vi "GUI_DG645_1.0.0.vi"() -> ()   [LabVIEW 2020]
uses:
  Device Drivers/DG645/subVIs/TriggerSource_TypDef.ctl
  Device Drivers/DG645/subVIs/Inhibit_TypDef.ctl
  Device Drivers/shared/OnOffTypeDef.ctl
  Device Drivers/DG645/subVIs/polarity_TypDEf.ctl
  DelayControl_For Multiple Channels.ctl
  Device Drivers/DG645/subVIs/channels_TypDef.ctl
  DelayControl2.ctl
  Device Drivers/DG645/subVIs/saveLocal_TypDef.ctl
panel:
  in  "time to wait (TCP) 2":i32=10
  in  "plot":bool=TRUE
  out "ratio(h)":bool
  out "fixsize":bool
  in  "shotnumber":i32
  out "error (h)":bool
  out "Device Name (h)":string="StagingDG645 1"
  in  "Main Tap":T1(tab)
  in  "Delay.Ch T1":T2={"Channel"="T1", "Linked"=enum."T0", "Delay"=0.03} {"Delay" format="%+.12f"}
  in  "Delay.Ch T0":T2={"Channel"="T0", "Linked"=enum."T0", "Delay"=0.0} {"Delay" format="%+.12f"}
  in  "Delay.Ch H":T2={"Channel"="H", "Linked"=enum."G", "Delay"=0.03} {"Delay" format="%+.12f"}
  in  "Delay.Ch G":T2={"Channel"="G", "Linked"=enum."T0", "Delay"=0.0} {"Delay" format="%+.12f"}
  in  "Delay.Ch F":T2={"Channel"="F", "Linked"=enum."E", "Delay"=0.03} {"Delay" format="%+.12f"}
  in  "Delay.Ch E":T2={"Channel"="E", "Linked"=enum."T0", "Delay"=0.0} {"Delay" format="%+.12f"}
  in  "Delay.Ch D":T2={"Channel"="D", "Linked"=enum."C", "Delay"=0.03} {"Delay" format="%+.12f"}
  in  "Delay.Ch C":T2={"Channel"="C", "Linked"=enum."T0", "Delay"=0.0} {"Delay" format="%+.12f"}
  in  "Delay.Ch B":T2={"Channel"="B", "Linked"=enum."A", "Delay"=0.03} {"Delay" format="%+.12f"}
  in  "Amplitude.Ch AB":dbl=3.0 caption="Amplitude (V)"
  in  "Amplitude.Ch CD":dbl=4.0 caption="Amplitude (V)"
  in  "Amplitude.Ch EF":dbl=4.0 caption="Amplitude (V)"
  in  "Amplitude.Ch GH":dbl=4.0 caption="Amplitude (V)"
  in  "Amplitude.Ch T0":dbl=4.0 caption="Amplitude (V)"
  in  "Polarity.Ch AB":T5=enum."Positive" caption="Polarity"
  in  "Polarity.Ch CD":T5=enum."Positive" caption="Polarity"
  in  "Polarity.Ch EF":T5=enum."Positive" caption="Polarity"
  in  "Polarity.Ch GH":T5=enum."Positive" caption="Polarity"
  in  "Polarity.Ch T0":T5=enum."Positive" caption="Polarity"
  in  "Delay.Ch A":T2={"Channel"="A", "Linked"=enum."T0", "Delay"=0.0} {"Delay" format="%+.12f"}
  in  "Trigger.ExecuteSingleShot":T6
  out "Array":cluster{"Waveform Graph":dbl[]}[](array[cluster])
  out "local Port":u16=65427
  out "port or service name":u16=65426
  out "Remote Host":string="192.168.11.97"
  in  "timeout ms (slow resp)":i32=500
  in  "reset":bool
  out "image con closed":bool
  out "image \nconnection":bool
  out "image con closed 2":bool=TRUE
  out "All Devices (h)":string[](array[string])=["StagingDG645 1", "StagingDG645 2"]
  in  "time to wait (TCP)":i32=10
  out "error out":errorcluster
  out "connections (hidden)":variant[](array[variant])=[variant(refnum<k16> refnum), variant(refnum<k16> refnum)]
  in  "time to wait (main loop)":i32=10
  out "Data String":string="Amplitude.Ch AB,3.000000000000\r\nAmplitude.Ch CD,4.000000000000\r\nAmplitude.Ch EF,4.000000000000\r\nAmplitude.Ch GH,4.000000000000\r\nAmplitude.Ch T0,4.000000000000\r\nDelay.Ch A,0.000000000000\r\nDelay.Ch B,0.030000000000\r\nDelay.Ch C,0.000000000000\r\nDelay.Ch D,0.030000000000\r\nDelay.Ch E,0.000000000000\r\nDelay.Ch F,0.030000000000\r\nDelay.Ch G,0.000000000000\r\nDelay.Ch H,0.030000000000\r\nDelay.Ch T0,0.000000000000\r\nDelay.Ch T1,0.030000\r\nInhibit,Triggers\r\nLinked.Ch A,T0\r\nLinked.Ch B,A\r\nLinked.Ch C,T0\r\nLinked.Ch D,C\r\nLinked.Ch E,T0\r\nLinked.Ch F,E\r\nLinked.Ch G,T0\r\nLinked.Ch H,G\r\nLocalSavingPath,c:\\temp\r\nSave,off\r\nTrigger.ExecuteSingleShot,\r\nTrigger.Level,1.000000\r\nTrigger.Rate,10.000000\r\nTrigger.Source,External rising edges\r\ntimeout,0.000000\r\nPolarity.Ch AB,Positive\r\nPolarity.Ch CD,Positive\r\nPolarity.Ch EF,Positive\r\nPolarity.Ch GH,Positive\r\nPolarity.Ch T0,Positive\r\n"
  out "data out":string="Cam1>>ScanStart>>no error,>>"
  in  "send":bool
  in  "send command":string="ScanStart>>Cam1only.txt"
  out "error 2":bool
  out "error message 2":string
  in  "Local Saving Path":path
  in  "Trigger.Rate":dbl=10.0 caption="Rate (Hz)"
  in  "Trigger.Source":T7=enum."External rising edges" caption="Source"
  in  "Inhibit":T8=enum."Triggers"
  in  "Trigger":bool
  in  "Save":bool caption="Save File"
  in  "Load File":bool
  in  "Load Local":T9
  in  "Save Local":T9
  out "stop":bool
  out "error message":string
  out "Data Connection out":bool=TRUE
  # "AB"
  # "CD"
  # "EF"
  # "GH"
  # "T0"
  # "="
  # "="
  # "="
  # "="
  # "="
  # "="
  # "="
  # "="
  # "="
  # "="
  # "TRIGGER"
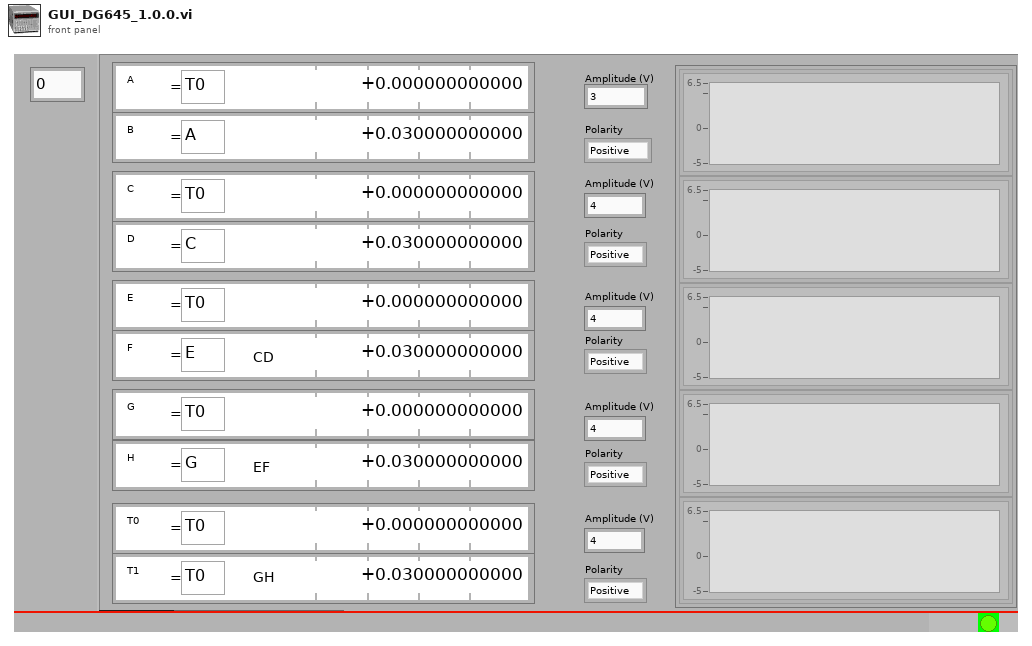
[diagram p1: front panel]
types:
  T1 = enum32{"All Channels", "Network", "Internal", "Advanced"}
  T2 = typedef "DelayControl_For Multiple Channels.ctl" = cluster{"Channel":string, "Linked":T3, "Delay":T4}
  T3 = typedef "channels_TypDef.ctl" = enum16{"T0", "T1", "A", "B", "C", "D", "E", "F", "G", "H"}
  T4 = typedef "DelayControl2.ctl" = dbl
  T5 = typedef "polarity_TypDEf.ctl" = enum16{"Negative", "Positive"}
  T6 = typedef "OnOffTypeDef.ctl" = enum16{"off", "on"}
  T7 = typedef "TriggerSource_TypDef.ctl" = enum16{"Internal", "External rising edges", "External falling edges", "Single shot external rising edges", "Single shot external falling edges", "Single shot", "Line"}
  T8 = typedef "Inhibit_TypDef.ctl" = enum16{"off", "Triggers", "AB", "AB and CD", "AB, CD and EF", "AB, CD, EF and GH"}
  T9 = typedef "saveLocal_TypDef.ctl" = enum16{"off", "1", "2", "3", "4", "5", "6", "7", "8", "9"}
  T10 = typedef "Type Descriptor__ogtk.ctl" = i16[]
  T11 = typedef "Type Descriptor Enumeration__ogtk.ctl" = enum8{"<Null>", "I8", "I16", "I32", "I64", "U8", "U16", "U32", "U64", "SGL", "DBL", "EXT", "CSG", "CDB", "CXT", "0x0F", "0x10", "0x11", "0x12", "0x13", "0x14", "Enum U8", "Enum U16", "Enum U32", "Enum U64", "SGL PQ", "DBL PQ", "EXT PQ", "CSG PQ", "CDB PQ", "CXT PQ", "0x1F", "0x20", "Boolean", "0x22", "0x23", "0x24", "0x25", "0x26", "0x27", "0x28", "0x29", "0x2A", "0x2B", "0x2C", "0x2D", "0x2E", "0x2F", "String", "0x31", "Path", "Pict", "0x34", "0x35", "0x36", "DAQ", "0x38", "0x39", "0x3A", "0x3B", "0x3C", "0x3D", "0x3E", "0x3F", "Array", "0x41", "0x42", "0x43", "0x44", "0x45", "0x46", "0x47", "0x48", "0x49", "0x4A", "0x4B", "0x4C", "0x4D", "0x4E", "0x4F", "Cluster", "0x51", "0x52", "Variant", "Waveform", "0x55", "0x56", "0x57", "0x58", "0x59", "0x5A", "0x5B", "0x5C", "0x5D", "0x5E", "0x5F", "0x60", "0x61", "0x62", "0x63", "0x64", "0x65", "0x66", "0x67", "0x68", "0x69", "0x6A", "0x6B", "0x6C", "0x6D", "0x6E", "0x6F", "Refnum"}
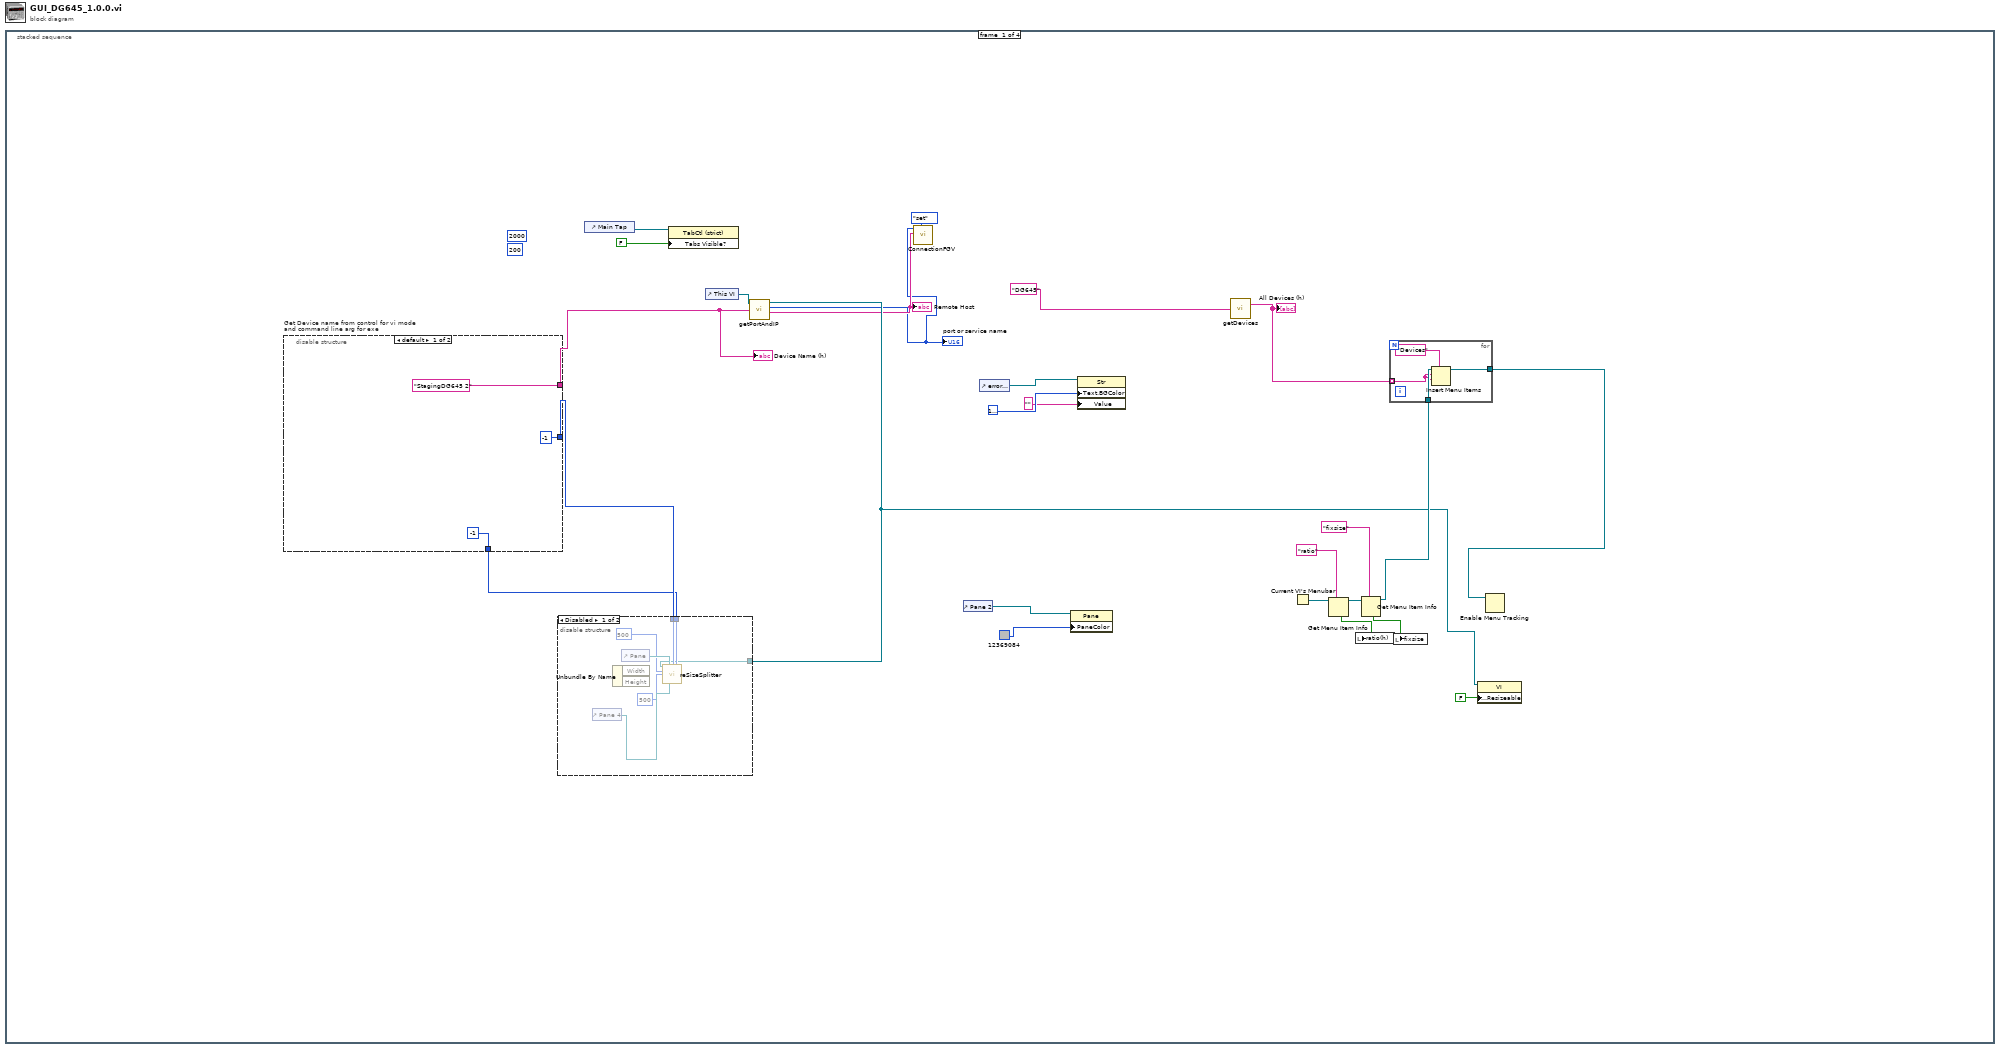
[diagram p0: block diagram]
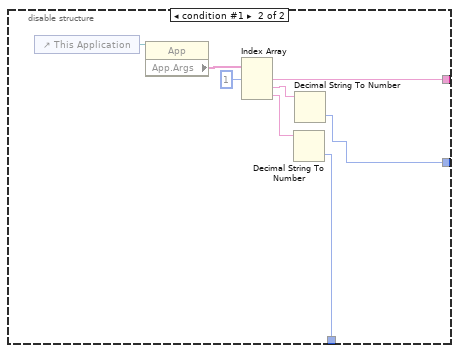
[diagram p3: hidden frame]
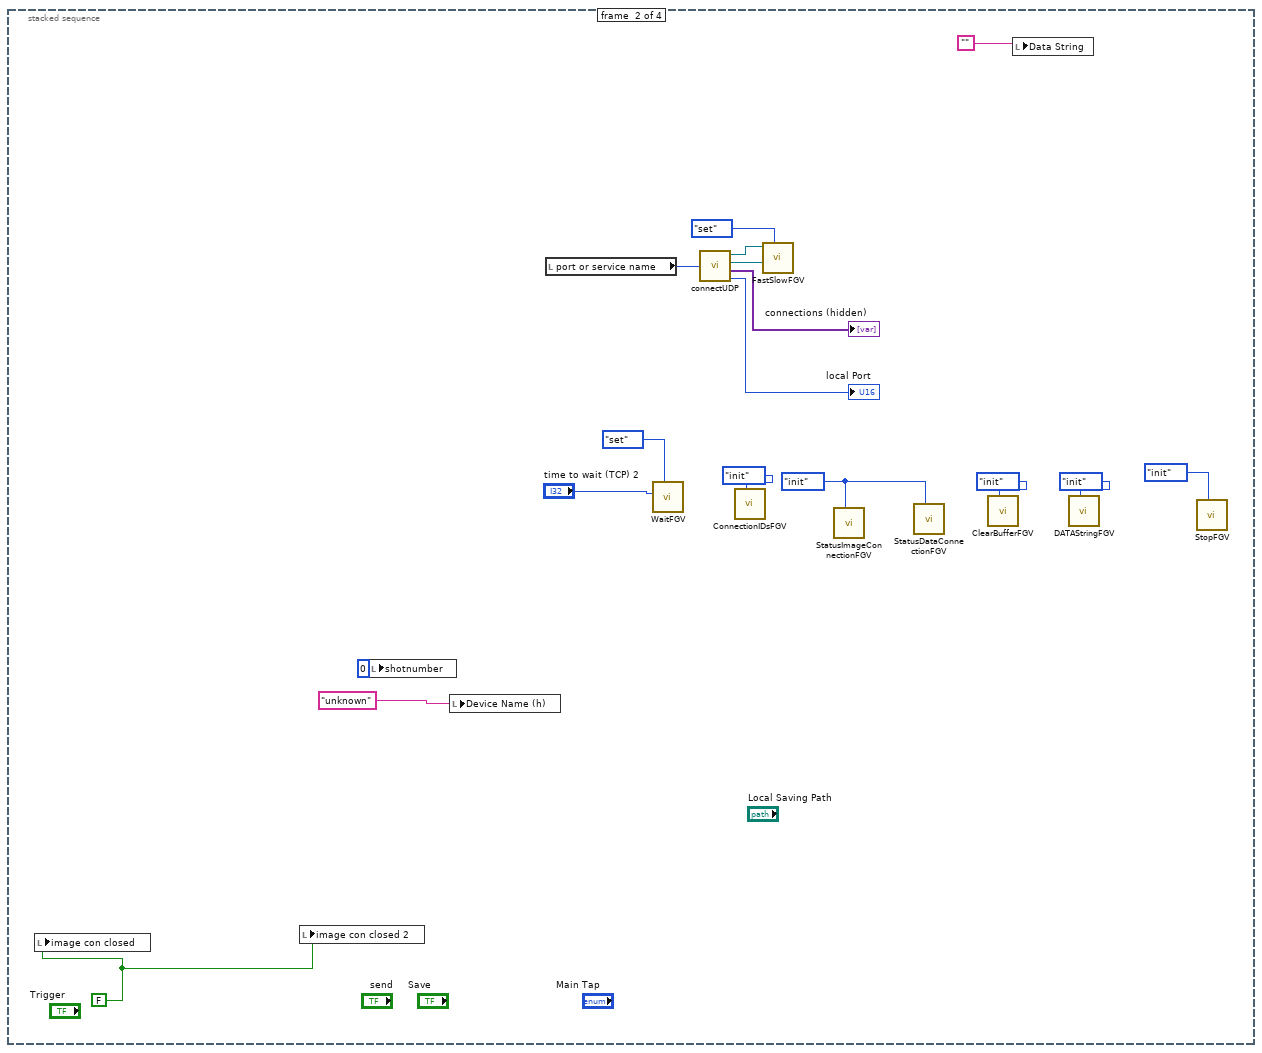
[diagram p4: hidden frame]
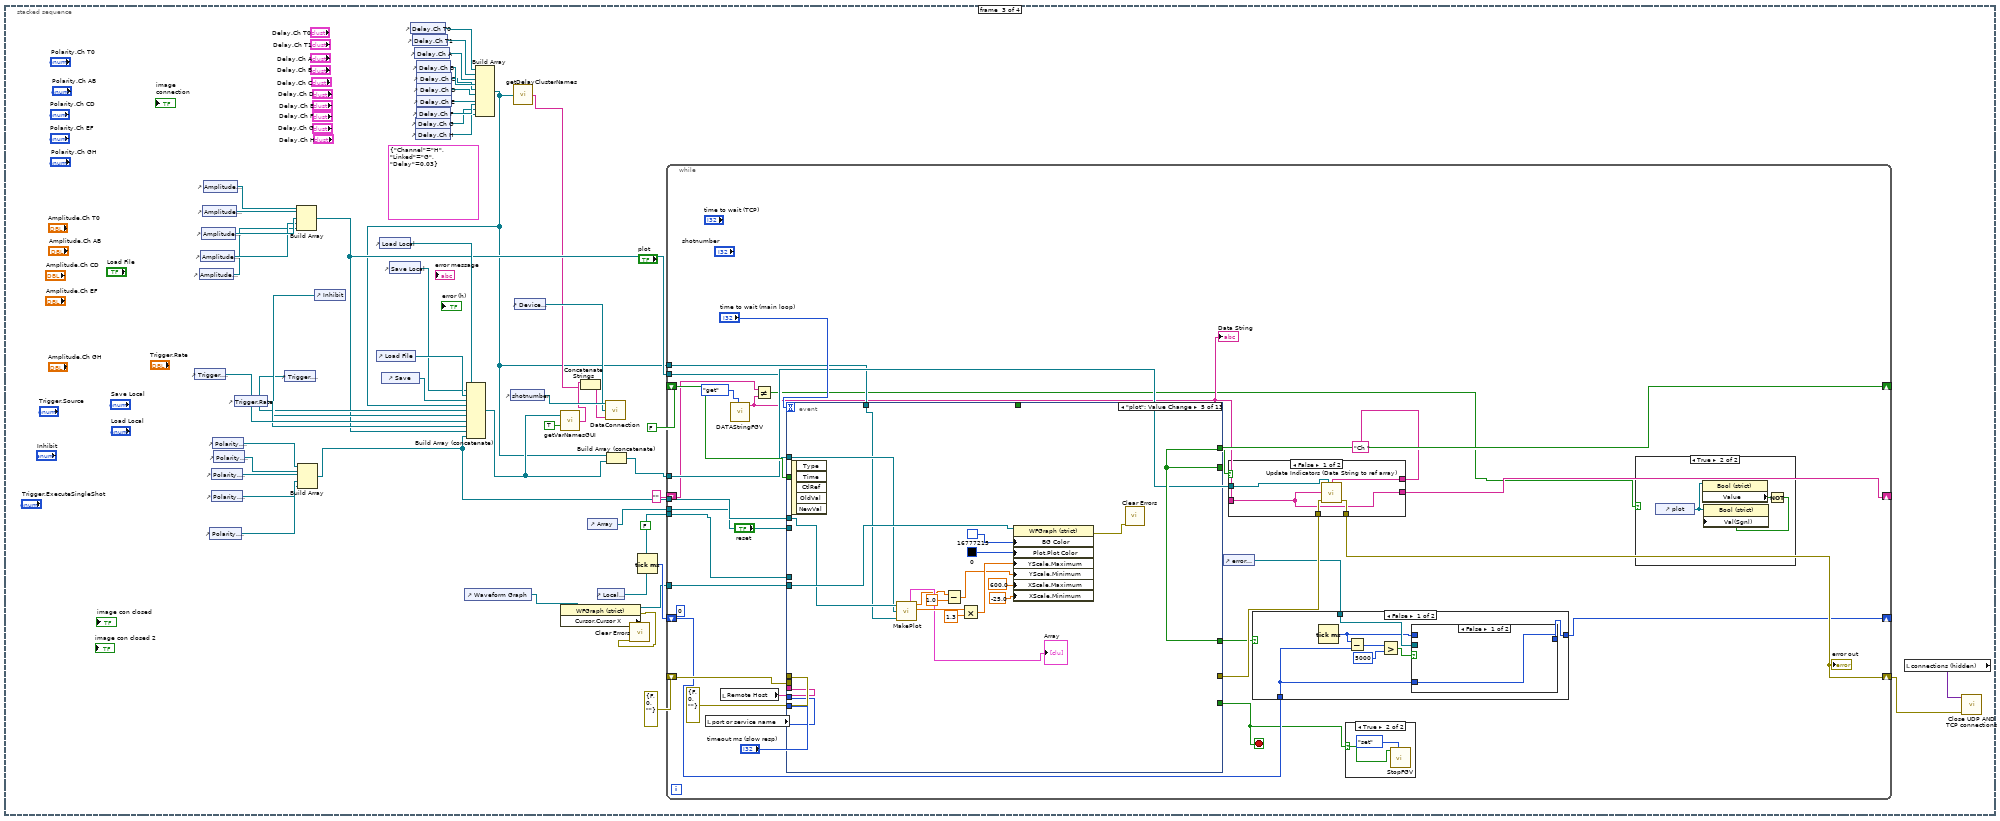
[diagram p5: hidden frame]
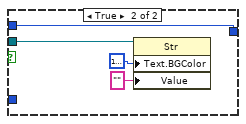
[diagram p8: hidden frame]
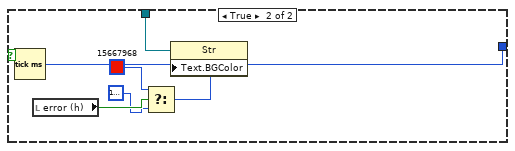
[diagram p9: hidden frame]
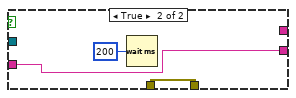
[diagram p10: hidden frame]
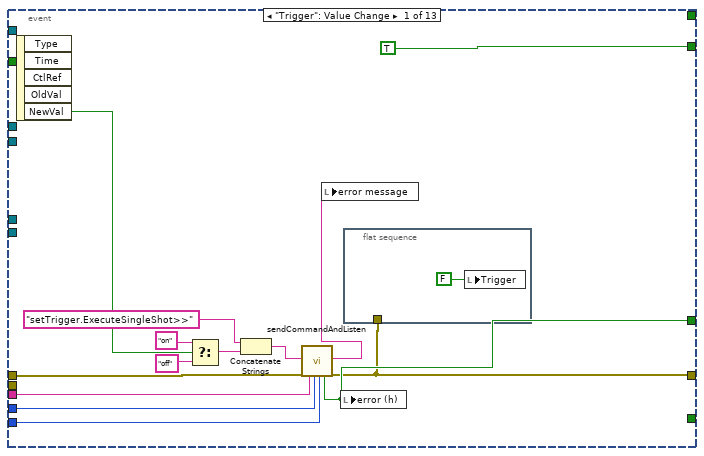
[diagram p11: hidden frame]
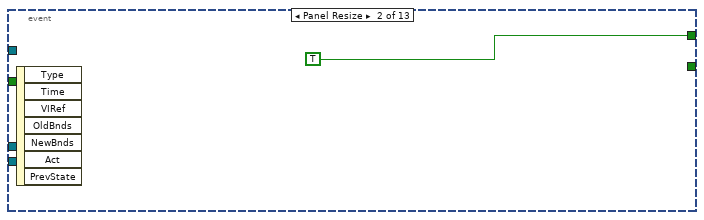
[diagram p12: hidden frame]
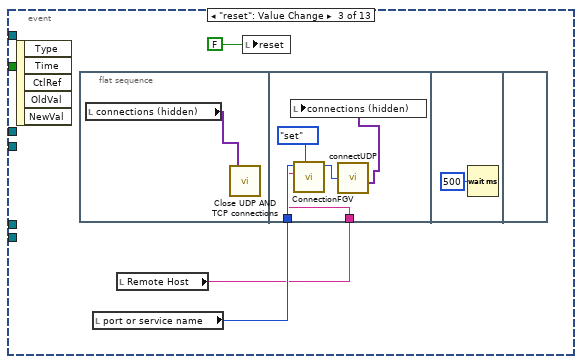
[diagram p13: hidden frame]
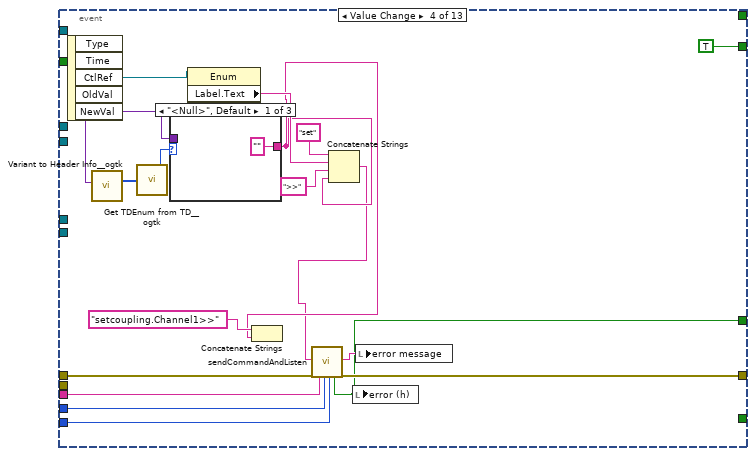
[diagram p14: hidden frame]
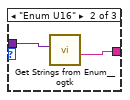
[diagram p15: hidden frame]
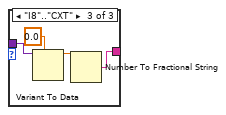
[diagram p16: hidden frame]
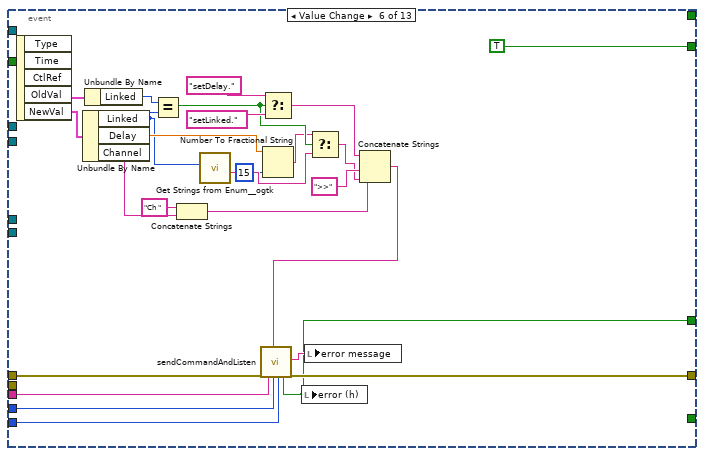
[diagram p17: hidden frame]
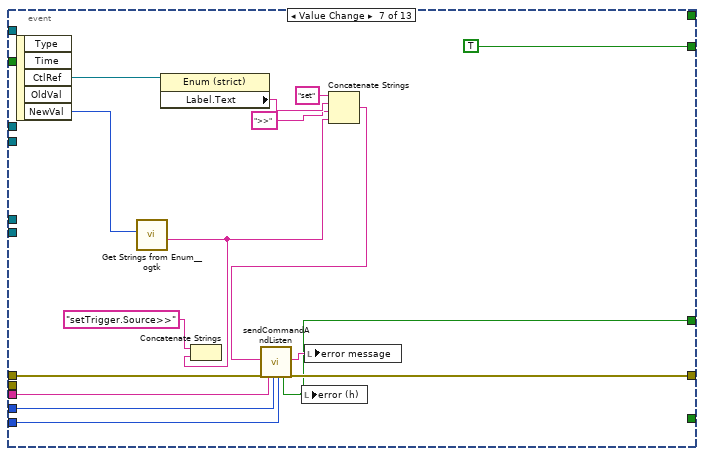
[diagram p18: hidden frame]
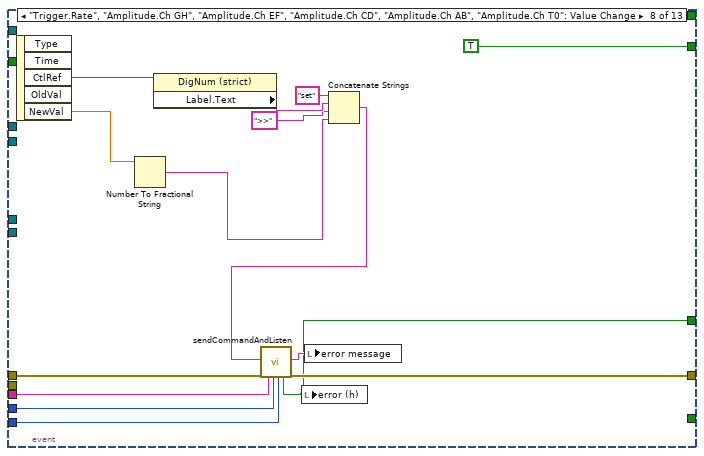
[diagram p19: hidden frame]
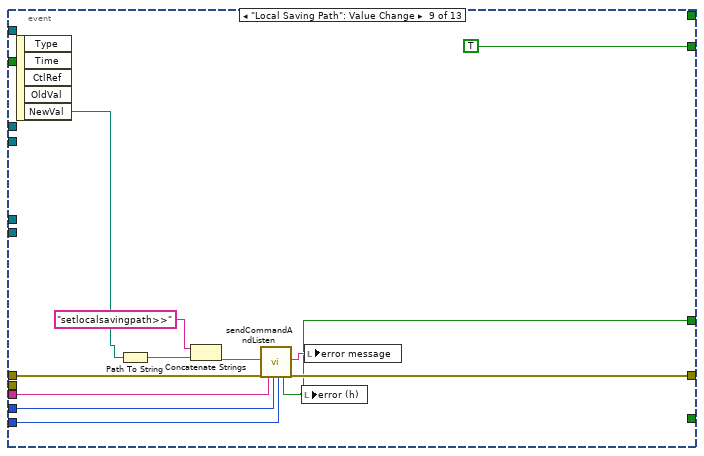
[diagram p20: hidden frame]
diagram:
  n1 = stacked-sequence {
    frame #0 {
      (unwired) i16 2000 ("Left")
      (unwired) i16 200 ("Top")
      n2 = disable-structure "Get Device name from control for vi mode\nand command line arg for exe" shown="default" {
        disable-tunnel: ["StagingDG645 2" ("Device Name for vi mode") w45] -> w8
        disable-tunnel: [i16 -1 ("left") w42] -> w19
        disable-tunnel: [i16 -1 ("left") w41] -> w18
        frame condition #0 (active) {
        }
        frame condition #1 {
          n3 = control-ref of="This Application"() -> (w48:refnum<vi>)
          n4 = property class="App"(reference=w48) -> ("App.Args"=w47:string[])  [unwired: 1 in, 2 out]
          n5 = Index Array(array=w47, index #1=1 ("index")) -> (element #1=w45:string, element #2=w44:string, element #3=w43:string)  [unwired: 2 in]
          n6 = Decimal String To Number(string=w43) -> (number=w41:i32)  [unwired: 2 in, 1 out]
          n7 = Decimal String To Number(string=w44) -> (number=w42:i32)  [unwired: 2 in, 1 out]
        }
      }
      "Device Name (h)" <- w8
      n8 = control-ref of="Main Tap"() -> (w26:refnum<vi>)
      n9 = property class="TabCtl (strict)"(reference=w26, "Tabs Visible?"=FALSE) -> ()  [unwired: 1 in, 2 out]
      n10 = control-ref of="This VI"() -> (w7:refnum<vi>)
      n11 = call "getPortAndIP.vi"("Device Name"=w8, "This Vi"=w7) -> ("Remote Host"=w2:string, "port or service name"=w1:u16, "reference out"=w4:refnum<vi>)  [unwired: 2 in, 2 out]
      "port or service name" <- w1
      "Remote Host" <- w2
      n12 = disable-structure shown="Disabled" {
        disable-tunnel: w19 -> [w32 _]
        disable-tunnel: w18 -> [w31 _]
        disable-tunnel: w4 -> [w29 _]
        frame Disabled {
          n13 = control-ref of="Pane 4"() -> (w30:refnum<vi>)
          n14 = Unbundle By Name() -> ()  [unwired: 1 in, 2 out]
          n15 = control-ref of="Pane"() -> (w33:refnum<vi>)
          n16 = call "reSizeSplitter.vi"("this vi"=w29, "pane"=w33, "left"=w32, "top"=w31, "Width"=u32 500, "Height"=u32 500, "pane2"=w30) -> ()  [unwired: 8 in, 1 out]
        }
        frame Enabled {
        }
      }
      n17 = call "ConnectionFGV.vi"("command"=enum16{"get", "set", "init"}."set", "Remote Host in"=w2, "port or service name in"=w1) -> ()  [unwired: 7 in, 2 out]
      n18 = control-ref of="Pane 2"() -> (w13:refnum<vi>)
      n19 = control-ref of="error message"() -> (w15:refnum<vi>)
      n20 = property class="Pane"(reference=w13, "PaneColor"=u32 12369084) -> ()  [unwired: 1 in, 2 out]
      n21 = property class="Str"(reference=w15, "Text.BGColor"=u32 16777238, "Value"="") -> ()  [unwired: 1 in, 2 out]
      n22 = call "getDevices.vi"("Device Class"="DG645") -> ("All Devices"=w9:string[])  [unwired: 1 out]
      "All Devices (h)" <- w9
      n23 = Current VI's Menubar() -> (w23:refnum<k9>)
      n24 = Get Menu Item Info(7:"ratio" ("item tag"), 11:w23) -> (3:w21:refnum<k9>, 4:w22:bool)  [unwired: 1 in, 5 out]
      n25 = local write "ratio(h)"(w22) -> ()
      n26 = Get Menu Item Info(7:"fixsize" ("item tag"), 11:w21) -> (3:w11:refnum<k9>, 4:w17:bool)  [unwired: 1 in, 5 out]
      n27 = for {
        tunnel: w11 -> [w37]
        tunnel: [w36] -> w10
        tunnel: w9 -> [w34] mode=indexing
        n28 = Insert Menu Items(5:"Devices" ("menu tag"), 7:w34, 8:w34, 9:w37) -> (3:w36:refnum<k9>)  [unwired: 2 in, 2 out]
      }
      n29 = local write "fixsize"(w17) -> ()
      n30 = property class="VI"(reference=w4, "Front Panel.Resizeable"=FALSE ("Front Panel Window:Resizable")) -> ()  [unwired: 1 in, 2 out]
      n31 = Enable Menu Tracking(4:w10) -> ()  [unwired: 2 in, 2 out]
    }
    frame #1 {
      w57 = enum16{"get", "set", "init"}."init" ("Command")
      w63 = FALSE ("new Device Data")
      n32 = local write "image con closed"(w63) -> ()
      n33 = local write "image con closed 2"(w63) -> ()
      n34 = local write "shotnumber"(0 ("shotnumber")) -> ()
      n35 = local write "Device Name (h)"("unknown" ("Device Name")) -> ()
      n36 = local read "port or service name"() -> (w53:u16)
      n37 = call "WaitFGV.vi"("Command"=enum16{"get", "set", "init"}."set", "milliseconds to wait"="time to wait (TCP) 2") -> ()  [unwired: 9 in, 1 out]
      n38 = call "connectUDP.vi"("port or service name NOT USED"=w53) -> ("fast ID (h)"=w52:refnum<k16>, "slow ID (h)"=w51:refnum<k16>, "connections (hidden)"=→"connections (hidden)":variant[], "local Port"=→"local Port":u16)
      n39 = call "ConnectionIDsFGV.vi"("Command"=enum16{"add", "get", "init"}."init") -> ()  [unwired: 10 in, 1 out]
      n40 = call "FastSlowFGV.vi"("Command"=enum16{"get", "set", "init"}."set", "slow ID"=w51, "fast ID"=w52) -> ()  [unwired: 7 in, 2 out]
      n41 = call "StatusImageConnectionFGV.vi"("Command"=w57) -> ()  [unwired: 10 in, 1 out]
      n42 = call "StatusDataConnectionFGV.vi"("Command"=w57) -> ()  [unwired: 10 in, 1 out]
      n43 = call "ClearBufferFGV.vi"("Command"=enum16{"set", "get", "init"}."init") -> ()  [unwired: 10 in, 1 out]
      n44 = local write "Data String"("") -> ()
      n45 = call "DATAStringFGV.vi"("Command"=enum16{"get", "set", "init"}."init") -> ()  [unwired: 9 in, 2 out]
      n46 = call "StopFGV.vi"("Command"=enum16{"set", "get", "init"}."init") -> ()  [unwired: 9 in, 2 out]
    }
    frame #2 {
      (unwired) T2 {"Channel"="H", "Linked"=enum."G", "Delay"=0.03} ("Delay.Ch H 2")
      (unwired) FALSE
      n47 = control-ref of="Trigger.Source"() -> (w109:refnum<vi>)
      n48 = control-ref of="Amplitude.Ch GH"() -> (w103:refnum<vi>)
      n49 = control-ref of="Amplitude.Ch EF"() -> (w104:refnum<vi>)
      n50 = control-ref of="Amplitude.Ch CD"() -> (w105:refnum<vi>)
      n51 = control-ref of="Amplitude.Ch AB"() -> (w106:refnum<vi>)
      n52 = control-ref of="Amplitude.Ch T0"() -> (w107:refnum<vi>)
      n53 = control-ref of="Polarity.Ch AB"() -> (w98:refnum<vi>)
      n54 = control-ref of="Polarity.Ch T0"() -> (w99:refnum<vi>)
      n55 = control-ref of="Polarity.Ch CD"() -> (w97:refnum<vi>)
      n56 = control-ref of="Polarity.Ch EF"() -> (w101:refnum<vi>)
      n57 = control-ref of="Polarity.Ch GH"() -> (w100:refnum<vi>)
      n58 = control-ref of="Trigger.Rate"() -> (w108:refnum<vi>)
      n59 = control-ref of="Trigger.ExecuteSingleShot"() -> (w86:refnum<vi>)
      n60 = Build Array(w107, w106, w105, w104, w103) -> (w80:refnum<vi>[])
      n61 = Build Array(w101, w100, w99, w98, w97) -> (w81:refnum<vi>[])
      n62 = control-ref of="Inhibit"() -> (w102:refnum<vi>)
      n63 = control-ref of="Load File"() -> (w84:refnum<vi>)
      n64 = control-ref of="Load Local"() -> (w83:refnum<vi>)
      n65 = control-ref of="Save"() -> (w85:refnum<vi>)
      n66 = control-ref of="Save Local"() -> (w82:refnum<vi>)
      n67 = control-ref of="Delay.Ch T0"() -> (w88:refnum<vi>)
      n68 = control-ref of="Delay.Ch T1"() -> (w87:refnum<vi>)
      n69 = control-ref of="Delay.Ch A"() -> (w96:refnum<vi>)
      n70 = control-ref of="Delay.Ch G"() -> (w90:refnum<vi>)
      n71 = control-ref of="Delay.Ch H"() -> (w89:refnum<vi>)
      n72 = control-ref of="Delay.Ch B"() -> (w95:refnum<vi>)
      n73 = control-ref of="Delay.Ch F"() -> (w91:refnum<vi>)
      n74 = control-ref of="Delay.Ch C"() -> (w94:refnum<vi>)
      n75 = control-ref of="Delay.Ch D"() -> (w93:refnum<vi>)
      n76 = control-ref of="Delay.Ch E"() -> (w92:refnum<vi>)
      n77 = control-ref of="Waveform Graph"() -> (w78:refnum<vi>)
      n78 = Build Array(w88, w87, w96, w95, w94, w93, w92, w91, w90, w89) -> (w66:refnum<vi>[])
      n79 = Build Array (concatenate)(w83, w82, w84, w85, w66, w86, w102, w109, w108, w80, w81) -> (w72:refnum<vi>[])
      n80 = control-ref of="shotnumber"() -> (w74:refnum<vi>)
      n81 = call "getDelayClusterNames.vi"("appended array"=w66) -> ("spreadsheet string"=w69:string)
      n82 = control-ref of="Device Name (h)"() -> (w73:refnum<vi>)
      n83 = call "getVarNamesGUI.vi"("start"=TRUE, "Array"=w72) -> ("String"=w70:string)
      n84 = property class="WFGraph (strict)" props=["Cursor", "Cursor X"](reference=w78) -> (reference out=w77:refnum<vi>, error out=w76:errorcluster)  [unwired: 1 in, 1 out]
      n85 = Concatenate Strings(w70, w69) -> (w68:string)
      n86 = control-ref of="Array"() -> (w79:refnum<vi>)
      n87 = control-ref of="Local Saving Path"() -> (w110:refnum<vi>)
      n88 = call "DataConnection.vi"("Subscriber list"=w68, "Device Name (h)"=w73, "shotnumber"=w74) -> ()
      n89 = Build Array (concatenate)(w66, w72) -> (w71:refnum<vi>[])
      n90 = call <vilib>:"Clear Errors.vi"("error in (no error)"=w76) -> ()  [unwired: 5 in, 2 out]
      n91 = Tick Count (ms)() -> (millisecond timer value=w111:u32)
      n92 = while {
        shift-right: [w136] -> w114
        shift-left: errorcluster {"status"=FALSE, "code"=0, "source"=""} ("error out") -> [w140]
        tunnel: w71 -> [w127]
        shift-right: [w134] -> _
        shift-left: FALSE -> [w135]
        shift-right: [w133] -> _
        shift-left: w111 -> [w132]
        tunnel: w110 -> [w129]
        tunnel: w81 -> [w126]
        tunnel: w80 -> [w125]
        tunnel: w66 -> [w124]
        tunnel: w79 -> [w123]
        tunnel: w77 -> [w122]
        shift-right: [w121] -> _
        shift-left: "" ("Data String") -> [w119]
        stop <- w116 stop-if-true
        (unwired) u32 0 ("Active Cursor")
        n93 = local read "port or service name"() -> (w138:u16)
        n94 = local read "Remote Host"() -> (w139:string)
        n95 = call "DATAStringFGV.vi"("Command"=enum16{"get", "set", "init"}."get") -> ("Data String out"=w118:string)  [unwired: 9 in, 1 out]
        "Data String" <- w118
        n96 = Not Equal?(x=w119, y=w118) -> (x != y?=w117:bool)
        n97 = event shown="[4] \"plot\": Value Change" {
          selector: _ -> [_ _ _ _ _ _ _ _ _ _ _ _ _]
          dyn-events: _ -> [_ _ _ _ _ _ _ _ _ _ _ _ _]
          timeout: "time to wait (main loop)" -> [_ _ _ _ _ _ _ _ _ _ _ _ _]
          tunnel: [w175 _ _ w217 _ w266 w281 w297 w307 w320 w335 w342 _] -> w137
          tunnel: errorcluster {"status"=FALSE, "code"=0, "source"=""} ("error out") -> [w179 _ _ w218 _ w267 w282 w298 w308 w321 w336 _ _]
          tunnel: w139 -> [w181 _ _ w216 _ w265 w280 w296 w306 w322 w334 _ _]
          tunnel: w138 -> [w182 _ _ w215 _ w264 w279 w295 w305 w319 w333 _ _]
          tunnel: "timeout ms (slow resp)" -> [w183 _ _ w214 _ w263 w278 w294 w304 w318 w332 _ _]
          tunnel: w140 -> [_ _ _ _ _ _ _ _ _ _ _ w342 _]
          tunnel: [TRUE _ _ TRUE _ TRUE TRUE TRUE TRUE TRUE TRUE _ _] -> w130
          tunnel: [_ _ _ _ _ _ _ _ _ _ _ _ w348] -> w116
          tunnel: [_ _ _ _ _ _ _ _ _ _ _ w341 w345] -> _
          tunnel: w135 -> [_ _ _ _ _ _ _ _ _ _ _ w341 _]
          tunnel: [_ TRUE _ _ _ _ _ _ _ _ _ _ _] -> w134
          tunnel: [w177 _ _ w211 _ w260 w275 w291 w299 w315 w328 _ _] -> _
          tunnel: w129 -> [_ _ _ _ _ _ _ _ _ _ _ _ w343]
          tunnel: w126 -> [_ _ _ _ w232 _ _ _ _ _ _ _ _]
          tunnel: w125 -> [_ _ _ _ w231 _ _ _ _ _ _ _ _]
          tunnel: w124 -> [_ _ _ _ w230 _ _ _ _ _ _ _ _]
          tunnel: w123 -> [_ _ _ _ _ _ _ _ _ _ _ _ _]
          tunnel: w122 -> [_ _ _ _ w233 _ _ _ _ _ _ _ _]
          event "Trigger": Value Change {
            n98 = event-data() -> ("NewVal"=w188:bool)  [unwired: 1 in, 4 out]
            n99 = Select(t="on", s=w188, f="off") -> (s? t:f=w184:string)
            n100 = Concatenate Strings("setTrigger.ExecuteSingleShot>>" ("data in"), w184) -> (w180:string)
            n101 = call "sendCommandAndListen.vi"("command in"=w180, "error in"=w179, "Remote Host"=w181, "port or service name"=w182, "timeout ms (100)"=w183) -> ("error"=w177:bool, "error message"=w176:string, "error out"=w175:errorcluster)  [unwired: 7 in, 5 out]
            n102 = local write "error message"(w176) -> ()
            n103 = local write "error (h)"(w177) -> ()
            n104 = flat-sequence {
              tunnel: w175 -> [_]
              frame #0 {
                n105 = local write "Trigger"(FALSE ("Trigger")) -> ()
              }
            }
          }
          event Panel Resize {
            n106 = event-data() -> ()  [unwired: 1 in, 7 out]
          }
          event "reset": Value Change {
            n107 = event-data() -> ()  [unwired: 1 in, 5 out]
            n108 = flat-sequence {
              tunnel: w192 -> [w196]
              tunnel: w191 -> [w195]
              frame #0 {
                n109 = local read "connections (hidden)"() -> (w194:variant[])
                n110 = call "Close UDP AND TCP connections.vi"("appended array"=w194) -> ()  [unwired: 7 in]
              }
              frame #1 {
                n111 = call "ConnectionFGV.vi"("command"=enum16{"get", "set", "init"}."set", "Remote Host in"=w195, "port or service name in"=w196) -> ("port or service name out"=w198:u16)  [unwired: 7 in, 1 out]
                n112 = call "connectUDP.vi"("port or service name NOT USED"=w198) -> ("connections (hidden)"=w197:variant[])  [unwired: 3 out]
                n113 = local write "connections (hidden)"(w197) -> ()
              }
              frame #2 {
                n114 = Wait (ms)(milliseconds to wait=u32 500) -> ()  [unwired: 1 out]
              }
              frame #3 {
              }
            }
            n115 = local read "port or service name"() -> (w192:u16)
            n116 = local read "Remote Host"() -> (w191:string)
            n117 = local write "reset"(FALSE ("reset")) -> ()
          }
          event Value Change {
            n118 = event-data() -> ("CtlRef"=w210:refnum<vi>, "NewVal"=w203:variant)  [unwired: 1 in, 3 out]
            n119 = call <userlib>:"Variant to Header Info__ogtk.vi"("Variant"=w203) -> ("Type Descriptor"=w202:T10)  [unwired: 3 in, 2 out]
            n120 = call <userlib>:"Get TDEnum from TD__ogtk.vi"("Type Descriptor"=w202) -> ("Type Descriptor Enumeration"=w201:T11)  [unwired: 4 in]
            n121 = case shown="\"<Null>\", Default" w201 {
              tunnel: ["" ("String Value") w221 w222] -> w205
              tunnel: w203 -> [_ w220 w225]
              frame "<Null>", Default {
              }
              frame "Enum U16" {
                n122 = call <userlib>:"Get Strings from Enum__ogtk.vi"("Enum"=w220) -> ("String Value"=w221:string)  [unwired: 7 in, 3 out]
              }
              frame "I8".."CXT" {
                n123 = Variant To Data(type=0.0, Variant=w225) -> (data=w223:dbl)  [unwired: 1 in, 1 out]
                n124 = Number To Fractional String(number=w223) -> (F-format string=w222:string)  [unwired: 3 in]
              }
            }
            n125 = property class="Enum"(reference=w210) -> ("Label.Text"=w208:string)  [unwired: 1 in, 2 out]
            n126 = Concatenate Strings("setcoupling.Channel1>>" ("data in"), w205) -> ()  [unwired: 1 out]
            n127 = Concatenate Strings("set", w208, ">>" ("string"), w205) -> (w204:string)
            n128 = call "sendCommandAndListen.vi"("command in"=w204, "error in"=w218, "Remote Host"=w216, "port or service name"=w215, "timeout ms (100)"=w214) -> ("error"=w211:bool, "error message"=w213:string, "error out"=w217:errorcluster)  [unwired: 7 in, 5 out]
            n129 = local write "error (h)"(w211) -> ()
            n130 = local write "error message"(w213) -> ()
          }
          event "plot": Value Change {
            n131 = event-data() -> ()  [unwired: 1 in, 5 out]
            n132 = call "MakePlot.vi"("Polarity array"=w232, "Amplitude array"=w231, "Channel array"=w230) -> ("min value"=w227:dbl, "Numeric 3"=w237:dbl, "Array"=→"Array":cluster{"Pulse Pattern":dbl[]}[])  [unwired: 2 out]
            n133 = Subtract(x=w227, y=1.0) -> (x-y=w226:dbl)
            n134 = Multiply(x=w237, y=1.3) -> (x*y=w239:dbl)
            n135 = property class="WFGraph (strict)"(reference=w233, "BG Color"=u32 16777215 ("Color"), "Plot.Plot Color"=u32 0 ("Color"), "YScale.Maximum"=w239, "YScale.Minimum"=w226, "XScale.Maximum"=600.0 ("X Scale.Range:Maximum"), "XScale.Minimum"=-25.0 ("X Scale.Range:Minimum")) -> (error out=w228:errorcluster)  [unwired: 1 in, 1 out]
            n136 = call <vilib>:"Clear Errors.vi"("error in (no error)"=w228) -> ()  [unwired: 5 in, 2 out]
          }
          event Value Change {
            n137 = event-data() -> ("OldVal"=w254:T2, "NewVal"=w255:T2)  [unwired: 1 in, 3 out]
            n138 = Unbundle By Name(w255) -> ("Linked"=w247:T3, "Delay"=w248:T4, "Channel"=w249:string)
            n139 = Unbundle By Name(w254) -> ("Linked"=w253:T3)
            n140 = Equal?(x=w253, y=w247) -> (x = y?=w246:bool)
            n141 = Concatenate Strings("Ch " ("string"), w249) -> (w256:string)
            n142 = call <userlib>:"Get Strings from Enum__ogtk.vi"("Enum"=w247) -> ("String Value"=w243:string)  [unwired: 7 in, 3 out]
            n143 = Select(t="setDelay.", s=w246, f="setLinked.") -> (s? t:f=w250:string)
            n144 = Number To Fractional String(number=w248, precision (6)=i16 15) -> (F-format string=w245:string)  [unwired: 2 in]
            n145 = Select(t=w245, s=w246, f=w243) -> (s? t:f=w244:string)
            n146 = Concatenate Strings(w250, w256, ">>" ("string"), w244) -> (w258:string)
            n147 = call "sendCommandAndListen.vi"("command in"=w258, "error in"=w267, "Remote Host"=w265, "port or service name"=w264, "timeout ms (100)"=w263) -> ("error"=w260:bool, "error message"=w262:string, "error out"=w266:errorcluster)  [unwired: 7 in, 5 out]
            n148 = local write "error (h)"(w260) -> ()
            n149 = local write "error message"(w262) -> ()
          }
          event Value Change {
            n150 = event-data() -> ("CtlRef"=w273:refnum<vi>, "NewVal"=w274:T7)  [unwired: 1 in, 3 out]
            n151 = call <userlib>:"Get Strings from Enum__ogtk.vi"("Enum"=w274) -> ("String Value"=w269:string)  [unwired: 7 in, 3 out]
            n152 = property class="Enum (strict)"(reference=w273) -> ("Label.Text"=w271:string)  [unwired: 1 in, 2 out]
            n153 = Concatenate Strings("setTrigger.Source>>" ("data in"), w269) -> ()  [unwired: 1 out]
            n154 = Concatenate Strings("set" ("string"), w271, ">>" ("string"), w269) -> (w268:string)
            n155 = call "sendCommandAndListen.vi"("command in"=w268, "error in"=w282, "Remote Host"=w280, "port or service name"=w279, "timeout ms (100)"=w278) -> ("error"=w275:bool, "error message"=w277:string, "error out"=w281:errorcluster)  [unwired: 7 in, 5 out]
            n156 = local write "error (h)"(w275) -> ()
            n157 = local write "error message"(w277) -> ()
          }
          event "Trigger.Rate", "Amplitude.Ch GH", "Amplitude.Ch EF", "Amplitude.Ch CD", "Amplitude.Ch AB", "Amplitude.Ch T0": Value Change {
            n158 = event-data() -> ("CtlRef"=w290:refnum<vi>, "NewVal"=w285:dbl)  [unwired: 1 in, 3 out]
            n159 = Number To Fractional String(number=w285) -> (F-format string=w284:string)  [unwired: 3 in]
            n160 = property class="DigNum (strict)"(reference=w290) -> ("Label.Text"=w288:string)  [unwired: 1 in, 2 out]
            n161 = Concatenate Strings("set" ("string"), w288, ">>" ("string"), w284) -> (w286:string)
            n162 = call "sendCommandAndListen.vi"("command in"=w286, "error in"=w298, "Remote Host"=w296, "port or service name"=w295, "timeout ms (100)"=w294) -> ("error"=w291:bool, "error message"=w293:string, "error out"=w297:errorcluster)  [unwired: 7 in, 5 out]
            n163 = local write "error (h)"(w291) -> ()
            n164 = local write "error message"(w293) -> ()
          }
          event "Local Saving Path": Value Change {
            n165 = event-data() -> ("NewVal"=w301:path)  [unwired: 1 in, 4 out]
            n166 = Path To String(path=w301) -> (string=w300:string)
            n167 = Concatenate Strings("setlocalsavingpath>>" ("data in"), w300) -> (w309:string)
            n168 = call "sendCommandAndListen.vi"("command in"=w309, "error in"=w308, "Remote Host"=w306, "port or service name"=w305, "timeout ms (100)"=w304) -> ("error"=w299:bool, "error message"=w303:string, "error out"=w307:errorcluster)  [unwired: 7 in, 5 out]
            n169 = local write "error (h)"(w299) -> ()
            n170 = local write "error message"(w303) -> ()
          }
          event "Save", "Load File": Value Change {
            n171 = event-data() -> ("CtlRef"=w314:refnum<vi>, "NewVal"=w327:bool)  [unwired: 1 in, 3 out]
            n172 = property class="Bool (strict)"(reference=w314) -> ("Label.Text"=w312:string)  [unwired: 1 in, 2 out]
            n173 = Select(t="on", s=w327, f="off") -> (s? t:f=w324:string)
            n174 = Concatenate Strings("set" ("data in"), w312, ">>" ("string"), w324) -> (w323:string)
            n175 = call "sendCommandAndListen.vi"("command in"=w323, "error in"=w321, "Remote Host"=w322, "port or service name"=w319, "timeout ms (100)"=w318) -> ("error"=w315:bool, "error message"=w317:string, "error out"=w320:errorcluster)  [unwired: 7 in, 5 out]
            n176 = local write "error (h)"(w315) -> ()
            n177 = local write "error message"(w317) -> ()
          }
          event "send": Value Change {
            n178 = event-data() -> ()  [unwired: 1 in, 5 out]
            n179 = local write "send"(FALSE ("sent")) -> ()
            n180 = call "sendCommandAndListen.vi"("command in"="send command", "error in"=w336, "Remote Host"=w334, "port or service name"=w333, "timeout ms (100)"=w332) -> ("error"=w328:bool, "error message"=→"error message 2":string, "data out"=→"data out":string, "error out"=w335:errorcluster)  [unwired: 7 in, 4 out]
            "error 2" <- w328
          }
          event Timeout {
            n181 = event-data() -> ()  [unwired: 1 in, 2 out]
            n182 = call "StatusDataConnectionFGV.vi"("Command"=enum16{"get", "set", "init"}."get") -> ("Data Connection out"=→"Data Connection out":bool)  [unwired: 10 in]
          }
          event Menu Selection (User) {
            n183 = event-data() -> ("MenuRef"=w344:refnum<k9>, "ItemTag"=w346:string)  [unwired: 1 in, 3 out]
            n184 = Equal?(x="Exit", y=w346) -> (x = y?=w348:bool)
            "stop" <- w348
            n185 = property on="Main Tap" class="TabCtl (strict)"() -> ("Value"=w350:T1)  [unwired: 2 in, 2 out]
            n186 = case shown="False" w348 {
              tunnel: w350 -> [w403 _]
              tunnel: w346 -> [w402 _]
              tunnel: [w399 errorcluster {"status"=FALSE, "code"=0, "source"=""} ("error out")] -> w347
              frame False {
                n187 = call <userlib>:"Set Enum String Value__ogtk.vi"("String Value"=w402, "Default Enum Value"=w403) -> ("error out"=w401:errorcluster, "Enum"=w405:variant)  [unwired: 8 in]
                n188 = Variant To Data(error in=w401, type=w403, Variant=w405) -> (data=w404:T1, error out=w400:errorcluster)
                n189 = property on="Main Tap" class="TabCtl (strict)"(error in=w400, "Value"=w404) -> (error out=w399:errorcluster)  [unwired: 1 in, 1 out]
              }
              frame True {
              }
            }
            n190 = case shown="Error" w347 {
              tunnel: w344 -> [_ w355]
              tunnel: w346 -> [_ w359]
              tunnel: [_ w360] -> w345
              tunnel: w343 -> [_ w353]
              frame No Error {
              }
              frame Error {
                n191 = local read "All Devices (h)"() -> (w357:string[])
                n192 = Get Menu Item Info(7:w359, 11:w355) -> (0:w356:errorcluster, 2:w362:string, 4:w363:bool)  [unwired: 1 in, 4 out]
                n193 = Not(x=w363) -> (.not. x?=w361:bool)
                n194 = Search 1D Array(1D array=w357, element=w359) -> (index of element=w358:i32)  [unwired: 1 in]
                n195 = Greater Or Equal To 0?(x=w358) -> (x >= 0?=w354:bool)
                n196 = case shown="True" w354 {
                  tunnel: w357 -> [_ w367]
                  tunnel: w356 -> [_ _]
                  tunnel: w355 -> [w364 w366]
                  tunnel: [w364 w365] -> w352
                  frame False {
                  }
                  frame True {
                    n197 = for {
                      tunnel: w367 -> [w371] mode=indexing
                      tunnel: w366 -> [w369]
                      tunnel: [w368] -> w365
                      n198 = Set Menu Item Info(6:FALSE ("checked"), 7:w371, 11:w369) -> (3:w368:refnum<k9>)  [unwired: 4 in, 1 out]
                    }
                  }
                }
                n199 = case shown="Default" w359 {
                  selector: w359 -> [_ w377 _ _ _ _]
                  tunnel: w361 -> [w372 w375 w386 _ _ _]
                  tunnel: [_ _ TRUE _ _ _] -> w360
                  tunnel: w354 -> [_ w378 _ _ _ _]
                  tunnel: w353 -> [_ _ _ w392 _ _]
                  tunnel: [w372 w376 w386 _ _ _] -> w351
                  frame "fixsize" {
                    n200 = control-ref of="This VI"() -> (w374:refnum<vi>)
                    n201 = Not(x=w372) -> (.not. x?=w373:bool)
                    n202 = property class="VI"(reference=w374, "Front Panel.Resizeable"=w373) -> ()  [unwired: 1 in, 2 out]
                    "fixsize" <- w372
                  }
                  frame Default {
                    n203 = case shown="True" w378 {
                      tunnel: w377 -> [_ w385]
                      tunnel: [_ w379] -> w376
                      tunnel: w375 -> [_ w379]
                      frame False {
                      }
                      frame True {
                        n204 = control-ref of="This VI"() -> (w384:refnum<vi>)
                        n205 = control-ref of="reset"() -> (w381:refnum<vi>)
                        n206 = call "getPortAndIP.vi"("Device Name"=w385, "This Vi"=w384) -> ("Remote Host"=w383:string, "port or service name"=w382:u16)  [unwired: 2 in, 3 out]
                        n207 = local write "port or service name"(w382) -> ()
                        n208 = local write "Remote Host"(w383) -> ()
                        n209 = property class="Bool (strict)"(reference=w381, "Val(Sgnl)"=TRUE ("Value (Signaling)")) -> ()  [unwired: 1 in, 2 out]
                      }
                    }
                  }
                  frame "ratio" {
                    "ratio(h)" <- w386
                  }
                  frame "Local Saving Path" {
                    n210 = property class="Path"(reference=w392) -> (reference out=w390:refnum<vi>, "Value"=w391:path)  [unwired: 1 in, 1 out]
                    n211 = call "changePath.vi"("Local Saving in (h)"=w391) -> ("change (h)"=w389:bool, "Local Saving out (h)"=w388:path)  [unwired: 9 in]
                    n212 = case shown="True" w389 {
                      tunnel: w390 -> [_ w394]
                      tunnel: w388 -> [_ w393]
                      frame False {
                      }
                      frame True {
                        n213 = property class="Path"(reference=w394, "Val(Sgnl)"=w393) -> ()  [unwired: 1 in, 2 out]
                      }
                    }
                  }
                  frame "reset" {
                    n214 = control-ref of="reset"() -> (w396:refnum<vi>)
                    n215 = property class="Bool (strict)"(reference=w396, "Val(Sgnl)"=TRUE ("Value (Signaling)")) -> ()  [unwired: 1 in, 2 out]
                  }
                  frame "clear" {
                    n216 = control-ref of="reset"() -> (w398:refnum<vi>)
                    n217 = property class="Bool (strict)"(reference=w398, "Val(Sgnl)"=TRUE ("Value (Signaling)")) -> ()  [unwired: 1 in, 2 out]
                  }
                }
                n218 = Set Menu Item Info(6:w351, 7:w359, 10:w362, 11:w352) -> ()  [unwired: 3 in, 2 out]
              }
            }
          }
        }
        n219 = control-ref of="error message"() -> (w131:refnum<vi>)
        n220 = case shown="False" w130 {
          tunnel: w127 -> [w169 _]
          tunnel: w137 -> [w168 w174]
          tunnel: [w171 w174] -> w136
          tunnel: "Ch " ("Channel Selector") -> [w170 _]
          tunnel: [w167 w172] -> w121
          tunnel: w118 -> [w167 w172]
          frame False {
            n221 = call "Update Indicators (Data String to ref array).vi"("Array"=w169, "Active Channel"=w170, "Data String"=w167, "error in (no error)"=w168) -> ("error out"=w171:errorcluster)  [unwired: 10 in, 1 out]
          }
          frame True {
            n222 = Wait (ms)(milliseconds to wait=u32 200) -> ()  [unwired: 1 out]
          }
        }
        "error out" <- w136
        n223 = case shown="False" w130 {
          tunnel: [w150 w166] -> w133
          tunnel: w132 -> [w149 _]
          tunnel: w131 -> [w152 w165]
          frame False {
            n224 = Tick Count (ms)() -> (millisecond timer value=w151:u32)
            n225 = Subtract(x=w151, y=w149) -> (x-y=w155:u32)
            n226 = Greater?(x=w155, y=u32 5000) -> (0:w153:bool)
            n227 = case shown="False" w153 {
              tunnel: w152 -> [_ w160]
              tunnel: w151 -> [_ w157]
              tunnel: [w156 w157] -> w150
              tunnel: w149 -> [w156 _]
              frame False {
              }
              frame True {
                n228 = property class="Str"(reference=w160, "Text.BGColor"=u32 16777238, "Value"="") -> ()  [unwired: 1 in, 2 out]
              }
            }
          }
          frame True {
            n229 = Tick Count (ms)() -> (millisecond timer value=w166:u32)
            n230 = local read "error (h)"() -> (w164:bool)
            n231 = Select(t=u32 15667968, s=w164, f=u32 16777238) -> (s? t:f=w161:u32)
            n232 = property class="Str"(reference=w165, "Text.BGColor"=w161) -> ()  [unwired: 1 in, 2 out]
          }
        }
        n233 = case shown="True" w116 {
          selector: w116 -> [_ w144]
          frame False {
          }
          frame True {
            n234 = call "StopFGV.vi"("Command"=enum16{"set", "get", "init"}."set", "Stop"=w144) -> ()  [unwired: 8 in, 2 out]
          }
        }
        n235 = case shown="True" w117 {
          frame False {
          }
          frame True {
            n236 = control-ref of="plot"() -> (w148:refnum<vi>)
            n237 = property class="Bool (strict)"(reference=w148) -> ("Value"=w147:bool)  [unwired: 1 in, 2 out]
            n238 = Not(x=w147) -> (.not. x?=w146:bool)
            n239 = property class="Bool (strict)"(reference=w148, "Val(Sgnl)"=w146) -> ()  [unwired: 1 in, 2 out]
          }
        }
      }
      n240 = local read "connections (hidden)"() -> (w113:variant[])
      n241 = call "Close UDP AND TCP connections.vi"("error in"=w114, "appended array"=w113) -> ()  [unwired: 6 in]
    }
    frame #3 {
      n242 = flat-sequence {
        frame #0 {
          n243 = Wait (ms)(milliseconds to wait=u32 0) -> ()  [unwired: 1 out]
        }
        frame #1 {
          n244 = local write "stop"(FALSE ("stop")) -> ()
        }
        frame #2 {
          n245 = control-ref of="This VI"() -> (w414:refnum<vi>)
          n246 = case shown="True" FALSE {
            tunnel: w414 -> [w415 w418]
            tunnel: [w415 w416] -> w413
            frame False {
            }
            frame True {
              n247 = property class="VI" props=["Front Panel.Open"](reference=w418) -> (reference out=w417:refnum<vi>)  [unwired: 1 in, 2 out]
              n248 = invoke class="VI" method="FP.Close"(reference=w417) -> (reference out=w416:refnum<vi>)  [unwired: 2 in, 2 out]
            }
          }
          n249 = Close Reference(reference=w413) -> ()  [unwired: 1 in, 1 out]
        }
      }
      n250 = control-ref of="Main  Control"() -> (w408:refnum<vi>)
      n251 = property class="TabCtl (strict)"(reference=w408, "Tabs Visible?"=TRUE) -> ()  [unwired: 1 in, 2 out]
      n252 = property class="TabCtl (strict)"(reference=w408, "Tab Location"=enum32{"Top", "Bottom", "Left", "Right"}."Bottom") -> ()  [unwired: 1 in, 2 out]
    }
  }
